vi "NetworkTest.vi"() -> ()   [LabVIEW 2014]
uses:
  <vilib>/Platform/TimedLoop/XDataNode/timing_clust.ctl
  <vilib>/Platform/TimedLoop/XDataNode/nitl_modes.ctl
  <vilib>/Platform/TimedLoop/XDataNode/wakeup.ctl
  <vilib>/Utility/tcp.llb/UDP Multicast Read-Write Open.vi
  <vilib>/platform/TimedLoop/XDataNode/XDataNode.xnode
  <vilib>/Platform/TimedLoop/XDataNode/XDNodeRunTimeDep.lvlib
  <vilib>/Utility/tcp.llb/UDP Multicast Read-Only Open.vi
panel:
  out "address":u32
  out "port":u16
  out "error out":errorcluster
  out "data out 2":string
  out "data out":string
  out "UDP_Out_Error Out 7":errorcluster
  out "UDP_Pack_num 7":u32
  out "UDP_Out Status 7":bool
  in  "Flight Number 5":string
  out "UDP_Out_Error Out 6":errorcluster
  out "UDP_Pack_num 6":u32
  out "UDP_Out Status 6":bool
  in  "Flight Number 4":string
  out "UDP_Out_Error Out 4":errorcluster
  out "UDP_Pack_num 4":u32
  out "UDP_Out Status 4":bool
  in  "Flight Number 3":string
  out "UDP_Out_Error Out 5":errorcluster
  out "UDP_Pack_num 5":u32
  out "UDP_Out Status 5":bool
  in  "Flight Number 2":string
  out "SEPTIC TCP Error Out 5":errorcluster
  out "TCP packet\nSend To SEPTIC 5":bool
  out "FISH TCP Error Out 5":errorcluster
  out "TCP packet\nSend To FISH 5":bool
  out "SEPTIC TCP Error Out 4":errorcluster
  out "TCP packet\nSend To SEPTIC 4":bool
  out "FISH TCP Error Out 4":errorcluster
  out "TCP packet\nSend To FISH 4":bool
  out "SEPTIC TCP Error Out 3":errorcluster
  out "TCP packet\nSend To SEPTIC 3":bool
  out "FISH TCP Error Out 3":errorcluster
  out "TCP packet\nSend To FISH 3":bool
  out "SEPTIC TCP Error Out 2":errorcluster
  out "TCP packet\nSend To SEPTIC 2":bool
  out "FISH TCP Error Out 2":errorcluster
  out "TCP packet\nSend To FISH 2":bool
  out "FISH TCP Error Out":errorcluster
  out "TCP packet\nSend To FISH":bool
  out "SEPTIC TCP Error Out":errorcluster
  out "TCP packet\nSend To SEPTIC":bool
  out "UDP_Pack_num 3":u32
  out "UDP_Out Status 3":bool
  out "UDP_Out_Error Out 3":errorcluster
  out "UDP_In":string
  out "UDP_In_Error":errorcluster
  in  "Flight Number":string
  in  "stop":bool
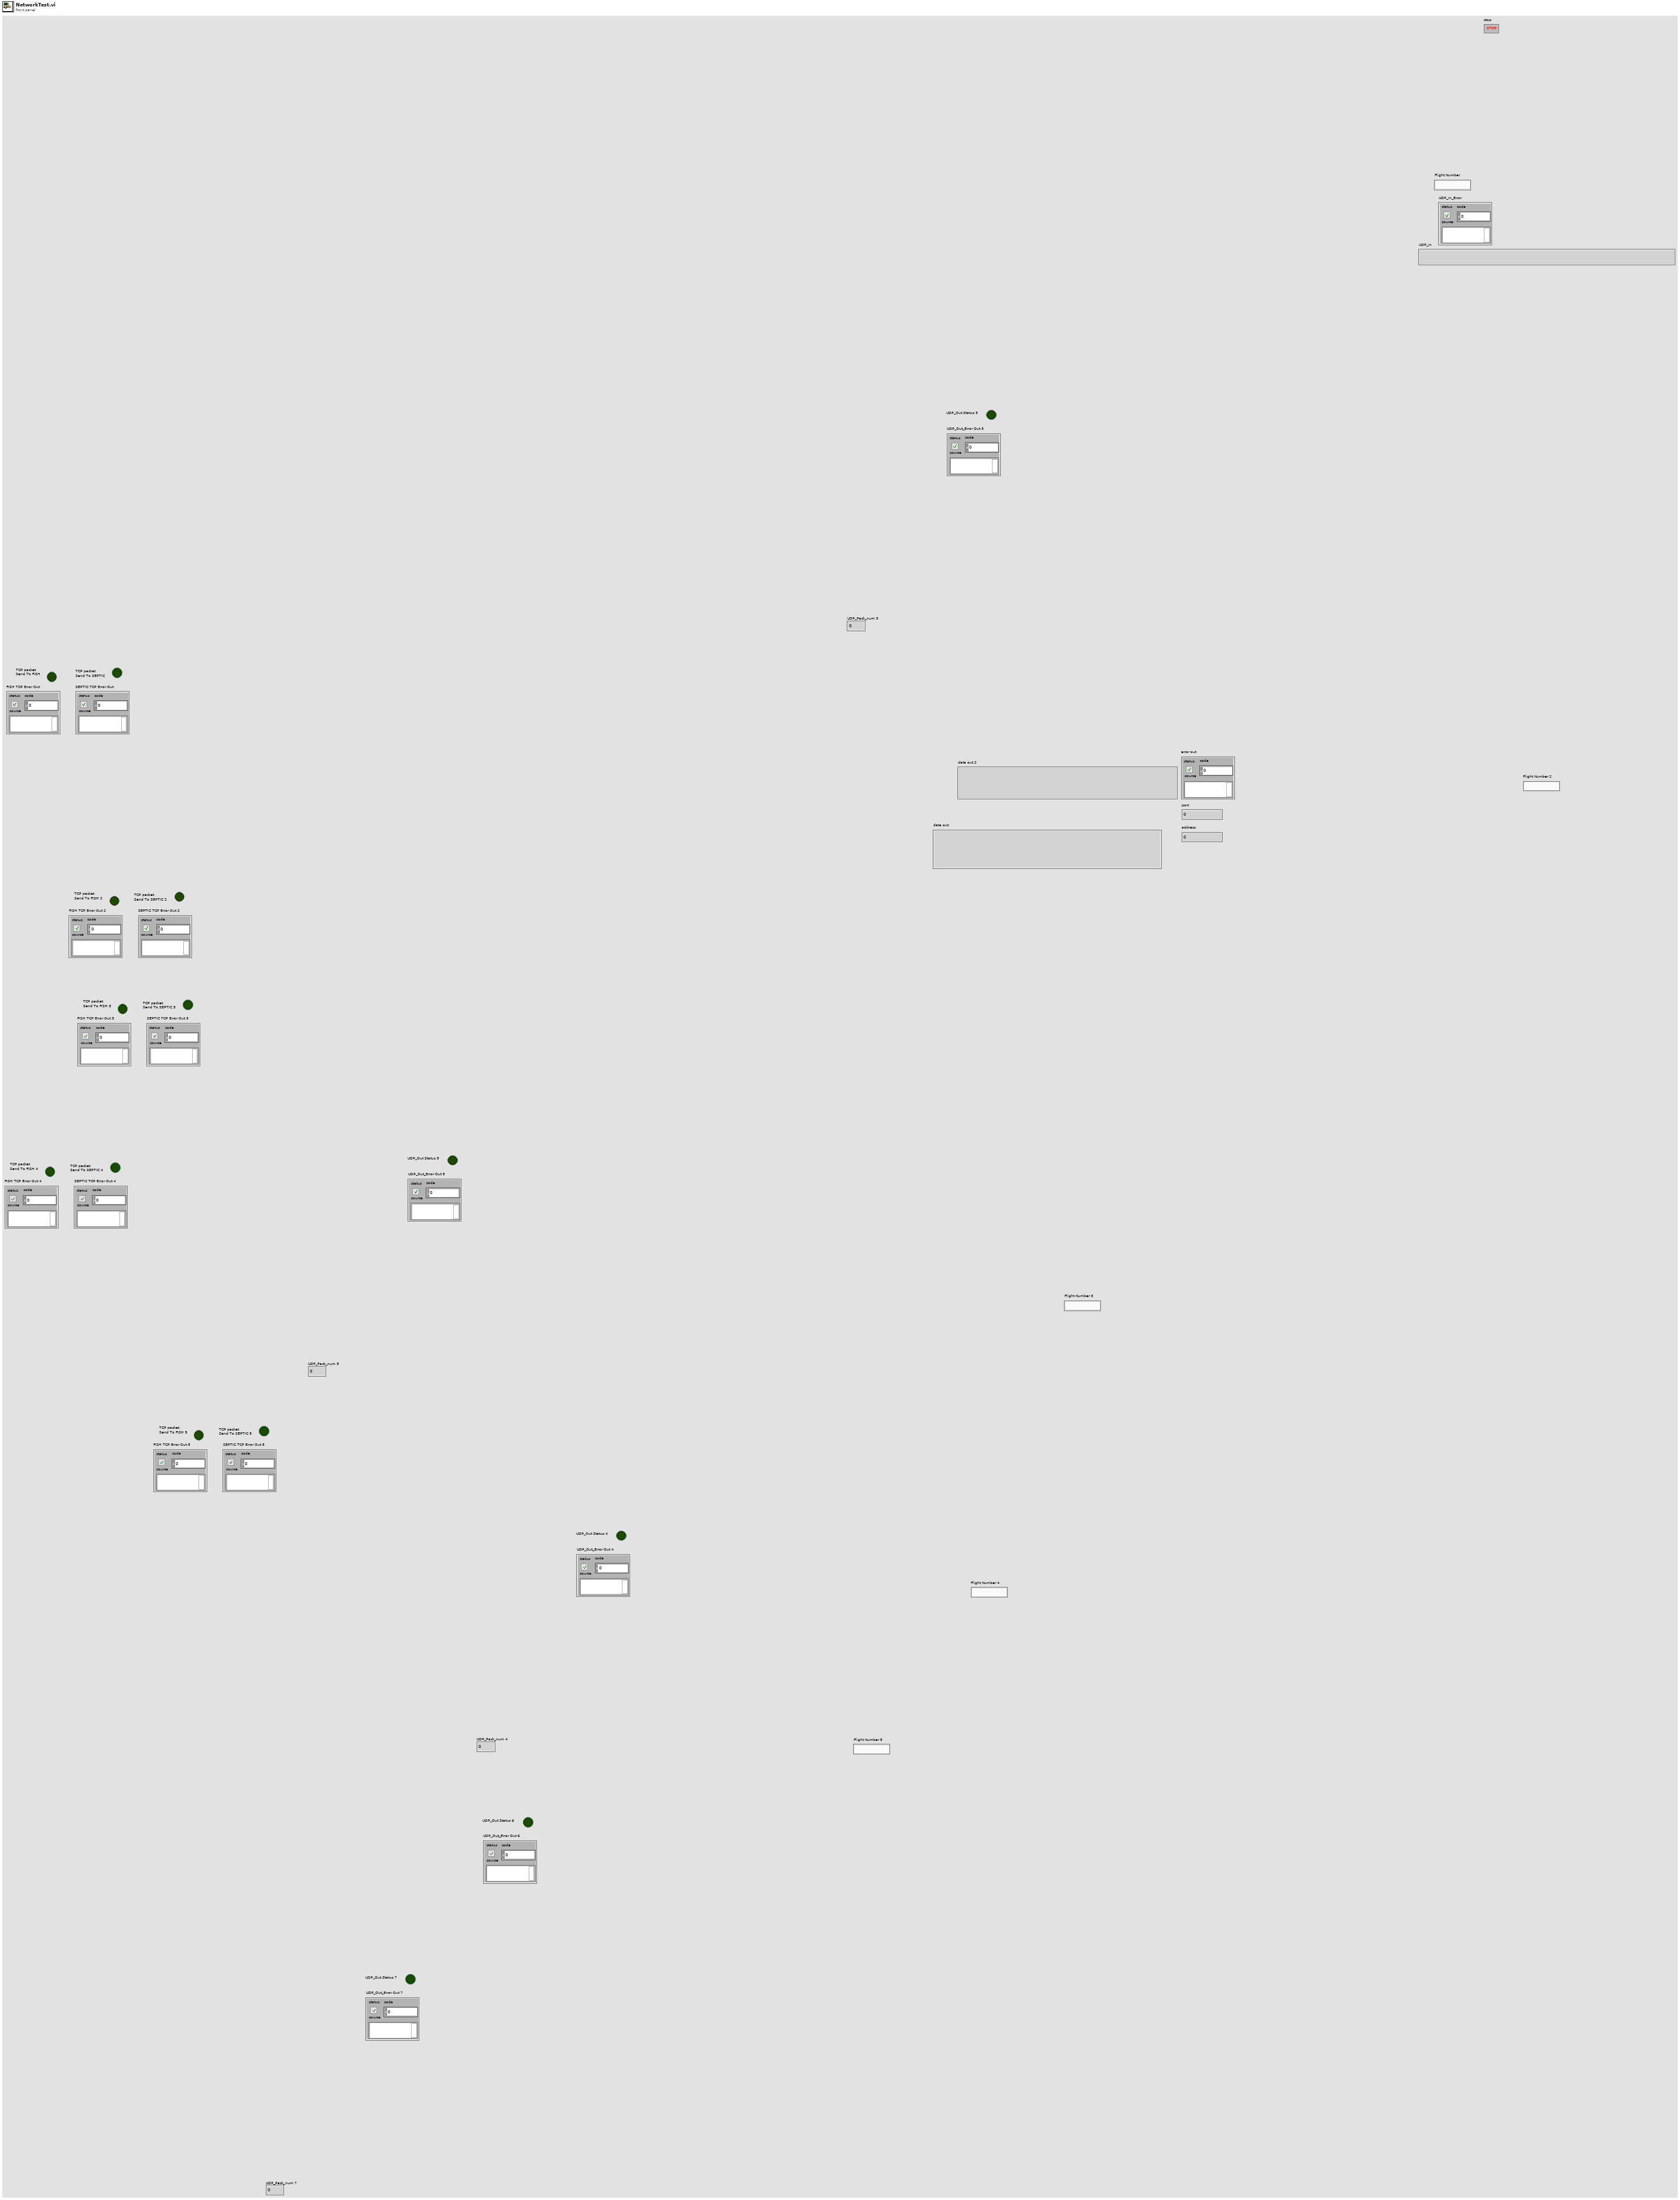
[diagram p1: front panel]
types:
  T1 = typedef "XDNodeRunTimeDep.lvlib/timing_clust.ctl" = cluster{"Expected End [f-1]":u64, "Actual End [f-1]":u64, "Finished Late? [f-1]":bool, "Expected End [i-1]":u64, "Actual End [i-1]":u64, "Finished Late? [i-1]":bool, "Expected Start [i]":u64, "Actual Start [i]":u64, "Expected Start [f]":u64, "Actual Start [f]":u64, "Source Name":string, "Structure Name":string, "Period":i64, "Deadline":i64, "Offset":i64, "Start":i64, "Priority":i32, "Timeout":i32, "Mode":T2, "Wakeup Reason":T3, "Error":errorcluster, "Source Type":string, "Secondary Source Type":string, "Global End Time":u64, "Global Start Time":u64, "Frame Duration":u64, "Iteration Duration":u64, "Assigned CPU":i32, "I/O Scan Engine Mode":u32}
  T2 = typedef "XDNodeRunTimeDep.lvlib/nitl_modes.ctl" = enum32{"No Change", "Process missed periods, maintain original phase", "Discard missed periods, maintain original phase", "Process missed periods, ignore original phase", "Discard missed periods, ignore original phase"}
  T3 = typedef "XDNodeRunTimeDep.lvlib/wakeup.ctl" = enum32{"Normal", "Aborted", "Asynchronous wakeup", "Timing source error", "Timed loop error", "Timeout"}
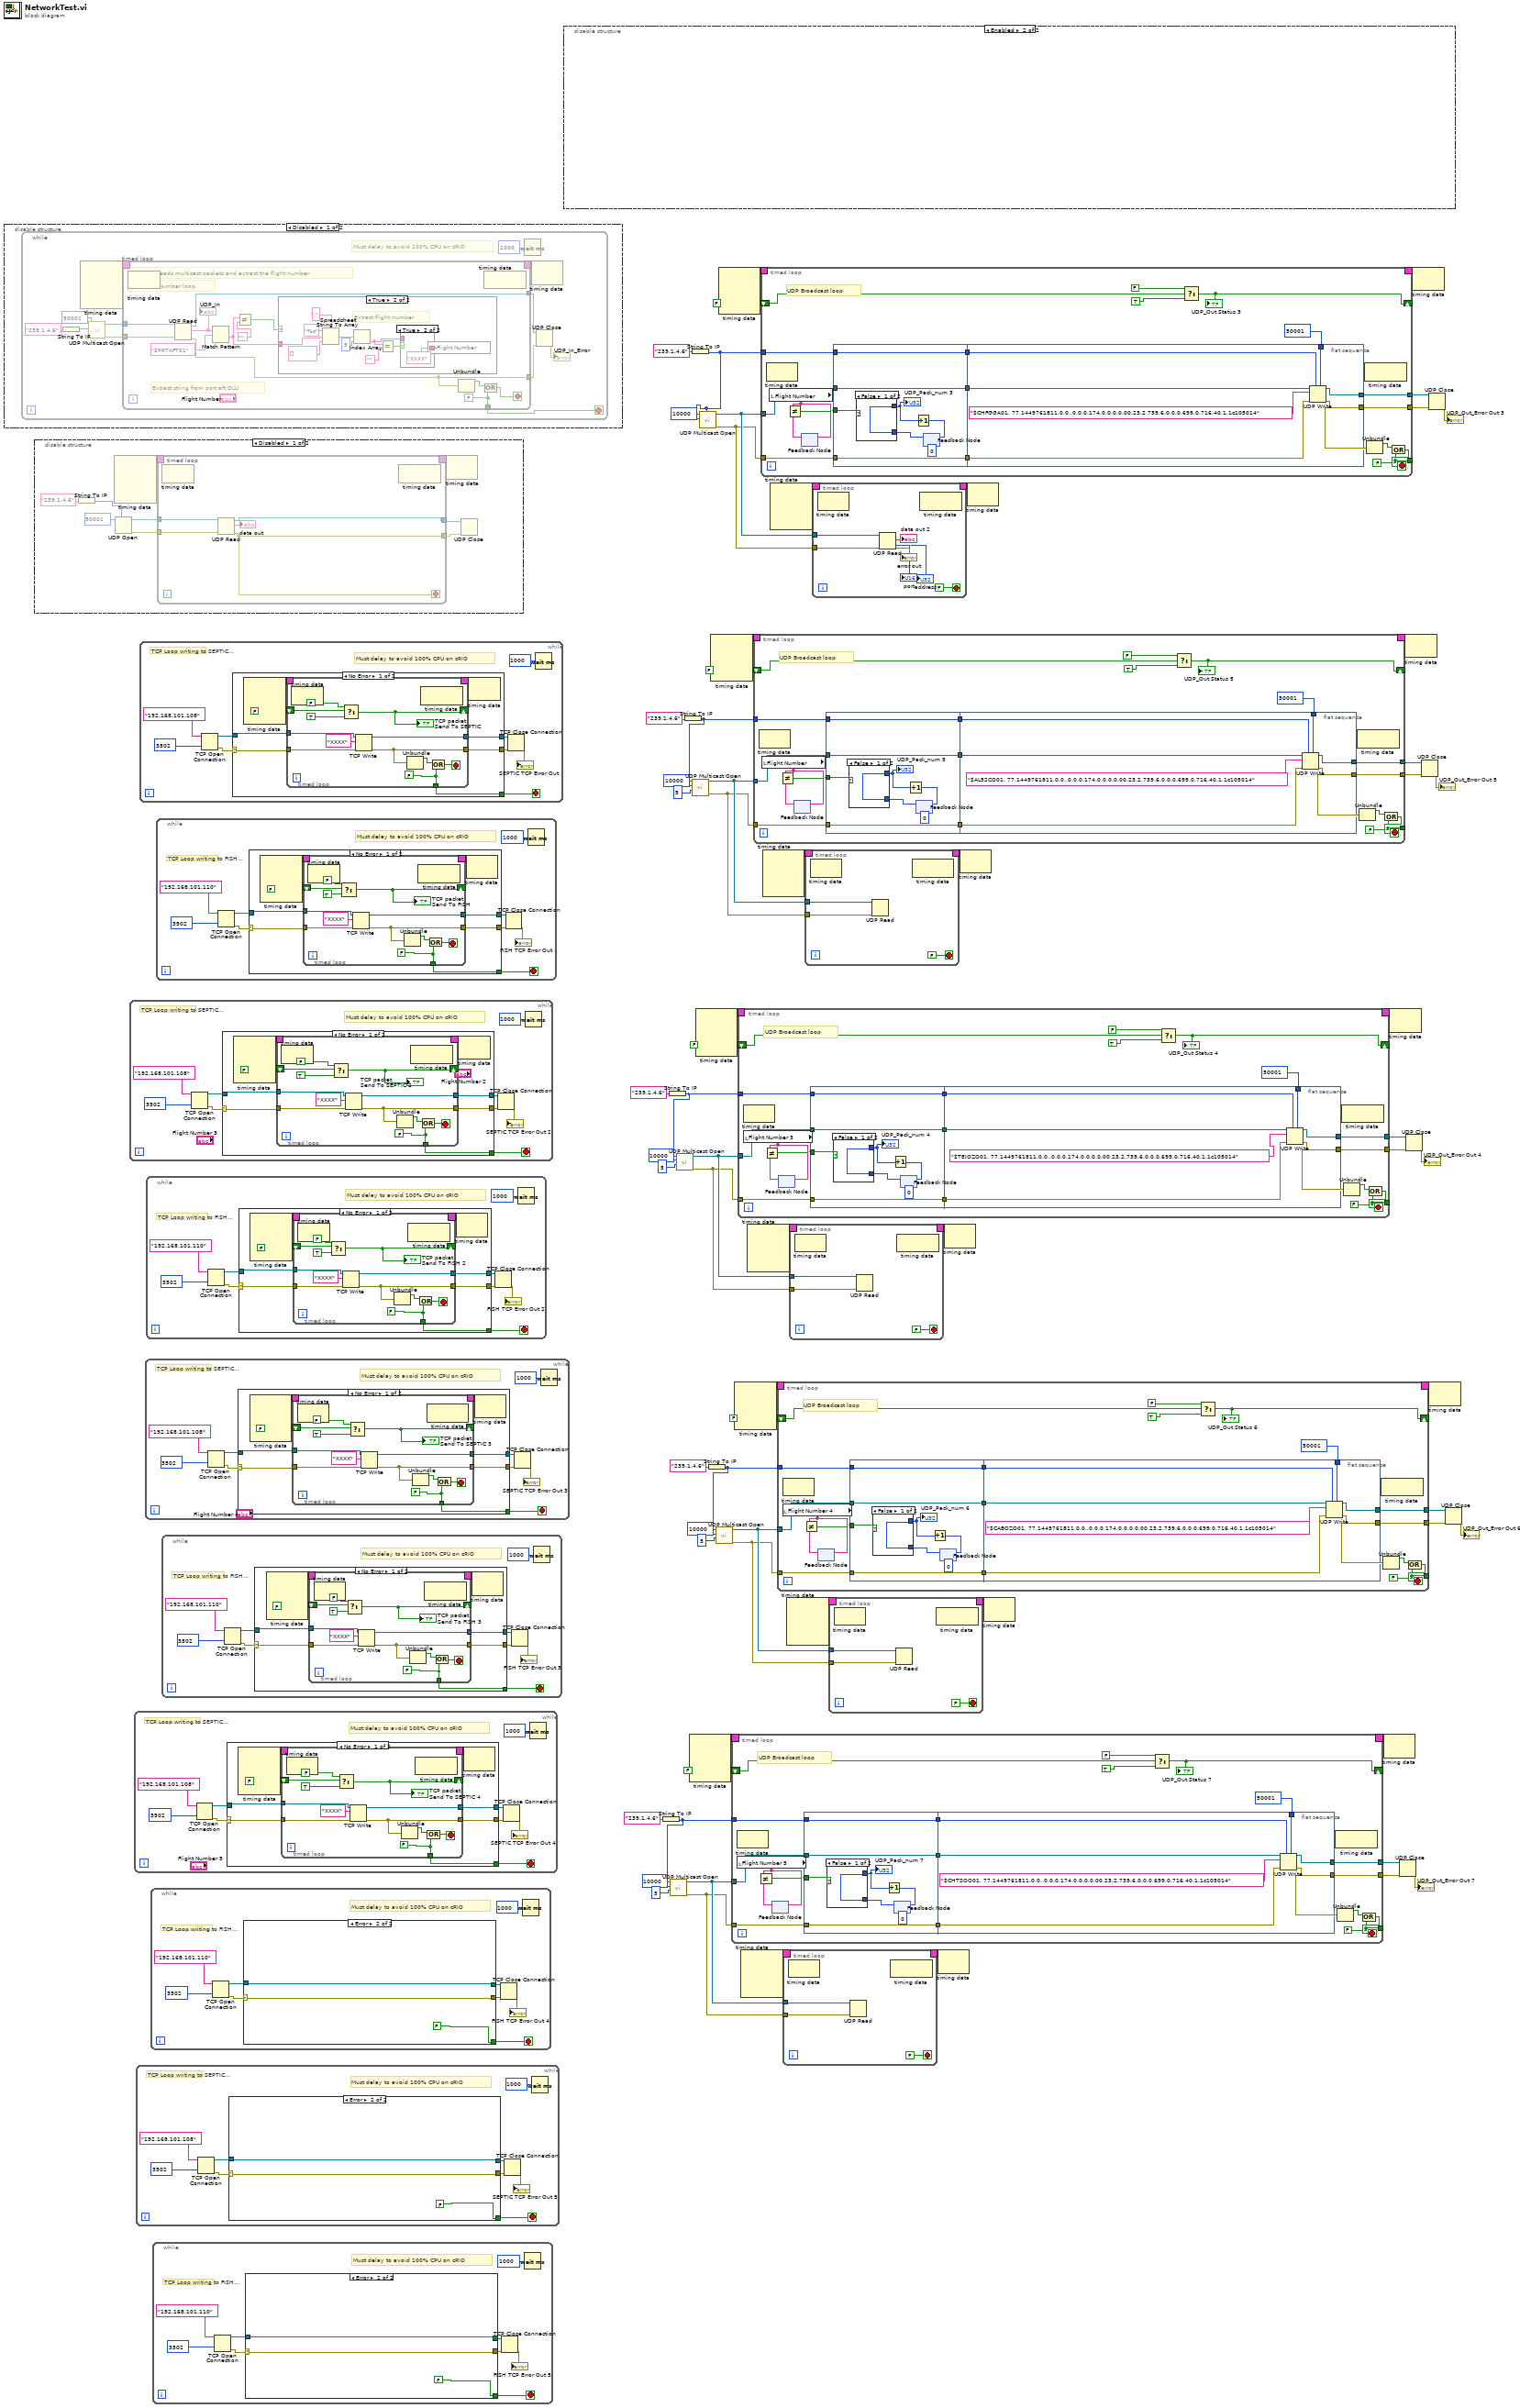
[diagram p0: block diagram]
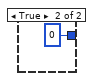
[diagram p6: hidden frame]
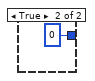
[diagram p7: hidden frame]
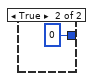
[diagram p8: hidden frame]
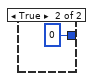
[diagram p9: hidden frame]
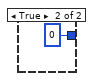
[diagram p10: hidden frame]
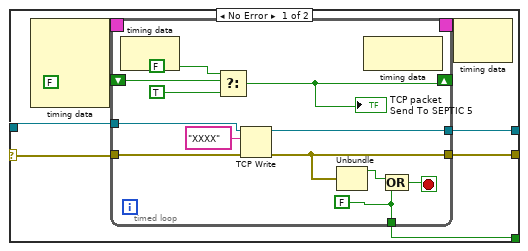
[diagram p11: hidden frame]
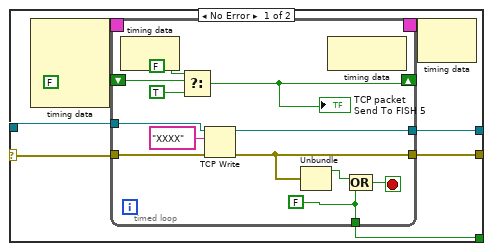
[diagram p12: hidden frame]
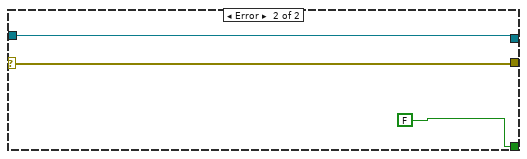
[diagram p13: hidden frame]
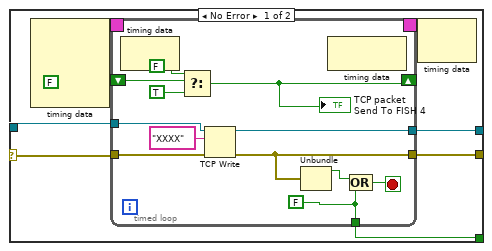
[diagram p14: hidden frame]
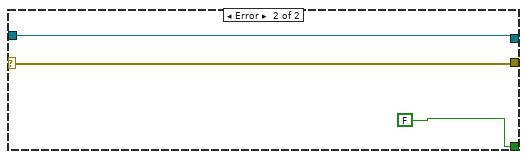
[diagram p15: hidden frame]
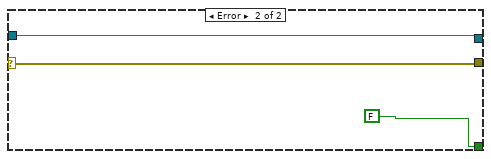
[diagram p16: hidden frame]
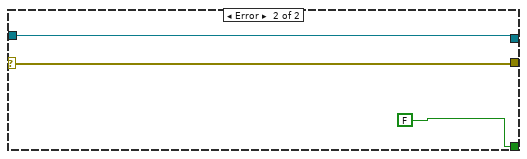
[diagram p17: hidden frame]
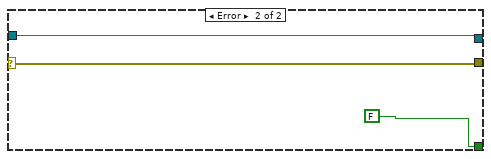
[diagram p18: hidden frame]
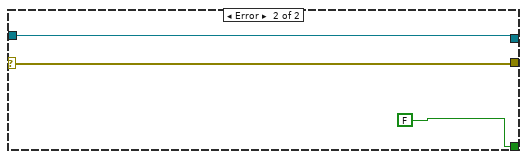
[diagram p19: hidden frame]
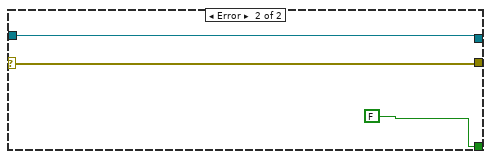
[diagram p20: hidden frame]
diagram:
  n1 = disable-structure shown="Disabled" {
    frame Disabled {
      n2 = while {
        stop <- w71 stop-if-true
        # "Must delay to avoid 100% CPU on cRIO"
        n3 = String To IP(1:"239.1.4.6" ("name")) -> (0:w79:u32)
        n4 = node-c288() -> (w81:T1)  [unwired: 4 in]
        n5 = call-poly <vilib>:"UDP Multicast Open.vi"("multicast addr"=w79, "port"=u16 50001) -> ("error out"=w75:errorcluster, "connection ID"=w76:refnum<k16>)  [unwired: 7 in, 1 out]
        n6 = timed-loop {
          tunnel: w76 -> [w93]
          tunnel: w75 -> [w92]
          timing: w81 -> [_]
          timing-out: [_] -> w80
          tunnel: [w86] -> w73
          tunnel: [w84] -> w72
          tunnel: [w82] -> w71
          stop <- w83 stop-if-true
          w82 = FALSE
          # "Extract string from port aft DLU"
          # "Get Flight Number loop"
          # "This loop reads multicast packets and extract the flight number"
          n7 = node-c288() -> ()  [unwired: 1 in, 1 out]
          n8 = UDP Read(connection ID=w93, 8:w92) -> (data out=w91:string, error out=w84:errorcluster, 3:w86:refnum<k16>)  [unwired: 2 in, 2 out]
          "UDP_In" <- w91
          n9 = Match Pattern(string=w91, regular expression="$PRTAFT01") -> (after substring=w87:string)  [unwired: 1 in, 3 out]
          n10 = Not Equal?(x=w87, y="") -> (x != y?=w88:bool)
          n11 = case shown="True" w88 {
            tunnel: w87 -> [_ w100]
            frame False {
            }
            frame True {
              # "Extract flight number"
              n12 = Spreadsheet String To Array(delimiter (Tab)=",", format string="%s", spreadsheet string=w100, array type (2D Dbl)=string[] []) -> (array=w102:string[])
              n13 = Index Array(array=w102, index=5) -> (element=w96:string)
              n14 = Equal?(x=w96, y="") -> (x = y?=w99:bool)
              n15 = case shown="True" w99 {
                tunnel: [w106 "XXXX"] -> w97
                tunnel: w96 -> [w106 _]
                frame False {
                }
                frame True {
                }
              }
              n16 = local write "Flight Number"(w97) -> ()
            }
          }
          n17 = Unbundle(w84) -> ("status"=w85:bool)  [unwired: 2 out]
          n18 = node-c288() -> ()  [unwired: 1 in, 1 out]
          n19 = Compound Arithmetic op=OR(w85, w82) -> (w83:bool)
        }
        n20 = Wait (ms)(milliseconds to wait=u32 1000) -> ()  [unwired: 1 out]
        n21 = node-c288(w80) -> ()  [unwired: 1 out]
        n22 = UDP Close(connection ID=w73, 8:w72) -> (error out=→"UDP_In_Error":errorcluster)  [unwired: 1 out]
      }
    }
    frame Enabled {
    }
  }
  n23 = disable-structure shown="Disabled" {
    frame Disabled {
      n24 = String To IP(1:"239.1.4.6" ("name")) -> (0:w110:u32)
      n25 = node-c288() -> (w118:T1)  [unwired: 4 in]
      n26 = UDP Open(7:w110, 11:u16 50001 ("port")) -> (port=w115:refnum<k16>, 0:w114:errorcluster)  [unwired: 3 in, 1 out]
      n27 = timed-loop {
        timing: w118 -> [_]
        timing-out: [_] -> w117
        tunnel: w115 -> [w123]
        tunnel: w114 -> [w122]
        tunnel: [w120] -> w112
        tunnel: [w119] -> w113
        stop <- w120 stop-if-true
        n28 = node-c288() -> ()  [unwired: 1 in, 1 out]
        n29 = UDP Read(connection ID=w123, 8:w122) -> (data out=→"data out":string, error out=w120:errorcluster, 3:w119:refnum<k16>)  [unwired: 2 in, 2 out]
        n30 = node-c288() -> ()  [unwired: 1 in, 1 out]
      }
      n31 = node-c288(w117) -> ()  [unwired: 1 out]
      n32 = UDP Close(connection ID=w113, 8:w112) -> ()  [unwired: 2 out]
    }
    frame Enabled {
    }
  }
  n33 = while {
    stop <- w131 stop-if-true
    # "Must delay to avoid 100% CPU on cRIO"
    # "TCP Loop writing to SEPTIC Tank"
    n34 = TCP Open Connection(address="192.168.101.108", remote port or service name=u16 3502) -> (connection ID=w134:refnum<k5>, error out=w129:errorcluster)  [unwired: 3 in]
    n35 = case shown="No Error" w129 {
      selector: w129 -> [w137 w162]
      tunnel: w134 -> [w142 w163]
      tunnel: [w141 w163] -> w133
      tunnel: [w140 w162] -> w132
      tunnel: [w139 FALSE] -> w131
      frame No Error {
        n36 = node-c288() -> (w144:T1)  [unwired: 4 in]
        n37 = timed-loop {
          tunnel: w142 -> [w156]
          tunnel: w137 -> [w155]
          tunnel: [w154] -> w141
          tunnel: [w153] -> w140
          tunnel: [w146] -> w139
          shift-right: [w147] -> _
          shift-left: FALSE -> [w150]
          timing: w144 -> [_]
          timing-out: [_] -> w143
          stop <- w151 stop-if-true
          w146 = FALSE
          n38 = node-c288() -> ()  [unwired: 1 in, 1 out]
          n39 = Select(t=FALSE, s=w150, f=TRUE) -> (s? t:f=w147:bool)
          "TCP packet\nSend To SEPTIC 2" <- w147
          n40 = TCP Write(connection ID=w156, data in="XXXX", error in (no error)=w155) -> (connection ID out=w154:refnum<k5>, error out=w153:errorcluster)  [unwired: 1 in, 1 out]
          n41 = Unbundle(w153) -> ("status"=w152:bool)  [unwired: 2 out]
          n42 = node-c288() -> ()  [unwired: 1 in, 1 out]
          n43 = Compound Arithmetic op=OR(w152, w146) -> (w151:bool)
        }
        n44 = node-c288(w143) -> ()  [unwired: 1 out]
      }
      frame Error {
      }
    }
    n45 = TCP Close Connection(connection ID=w133, error in (no error)=w132) -> (error out=→"SEPTIC TCP Error Out 2":errorcluster)  [unwired: 1 in, 1 out]
    n46 = Wait (ms)(milliseconds to wait=u32 1000) -> ()  [unwired: 1 out]
  }
  n47 = while {
    stop <- w167 stop-if-true
    # "Must delay to avoid 100% CPU on cRIO"
    # "TCP Loop writing to SEPTIC Tank"
    n48 = TCP Open Connection(address="192.168.101.108", remote port or service name=u16 3502) -> (connection ID=w170:refnum<k5>, error out=w165:errorcluster)  [unwired: 3 in]
    n49 = case shown="No Error" w165 {
      selector: w165 -> [w173 w198]
      tunnel: w170 -> [w178 w199]
      tunnel: [w177 w199] -> w169
      tunnel: [w176 w198] -> w168
      tunnel: [w175 FALSE] -> w167
      frame No Error {
        n50 = node-c288() -> (w180:T1)  [unwired: 4 in]
        n51 = timed-loop {
          tunnel: w178 -> [w192]
          tunnel: w173 -> [w191]
          tunnel: [w190] -> w177
          tunnel: [w189] -> w176
          tunnel: [w182] -> w175
          shift-right: [w183] -> _
          shift-left: FALSE -> [w186]
          timing: w180 -> [_]
          timing-out: [_] -> w179
          stop <- w187 stop-if-true
          w182 = FALSE
          n52 = node-c288() -> ()  [unwired: 1 in, 1 out]
          n53 = Select(t=FALSE, s=w186, f=TRUE) -> (s? t:f=w183:bool)
          "TCP packet\nSend To SEPTIC 4" <- w183
          n54 = TCP Write(connection ID=w192, data in="XXXX", error in (no error)=w191) -> (connection ID out=w190:refnum<k5>, error out=w189:errorcluster)  [unwired: 1 in, 1 out]
          n55 = Unbundle(w189) -> ("status"=w188:bool)  [unwired: 2 out]
          n56 = node-c288() -> ()  [unwired: 1 in, 1 out]
          n57 = Compound Arithmetic op=OR(w188, w182) -> (w187:bool)
        }
        n58 = node-c288(w179) -> ()  [unwired: 1 out]
      }
      frame Error {
      }
    }
    n59 = TCP Close Connection(connection ID=w169, error in (no error)=w168) -> (error out=→"SEPTIC TCP Error Out 4":errorcluster)  [unwired: 1 in, 1 out]
    n60 = Wait (ms)(milliseconds to wait=u32 1000) -> ()  [unwired: 1 out]
  }
  n61 = while {
    stop <- w203 stop-if-true
    # "Must delay to avoid 100% CPU on cRIO"
    # "TCP Loop writing to SEPTIC Tank"
    n62 = TCP Open Connection(address="192.168.101.108", remote port or service name=u16 3502) -> (connection ID=w206:refnum<k5>, error out=w201:errorcluster)  [unwired: 3 in]
    n63 = case shown="Error" w201 {
      selector: w201 -> [w209 w234]
      tunnel: w206 -> [w214 w235]
      tunnel: [w213 w235] -> w205
      tunnel: [w212 w234] -> w204
      tunnel: [w211 FALSE] -> w203
      frame No Error {
        n64 = node-c288() -> (w216:T1)  [unwired: 4 in]
        n65 = timed-loop {
          tunnel: w214 -> [w228]
          tunnel: w209 -> [w227]
          tunnel: [w226] -> w213
          tunnel: [w225] -> w212
          tunnel: [w218] -> w211
          shift-right: [w219] -> _
          shift-left: FALSE -> [w222]
          timing: w216 -> [_]
          timing-out: [_] -> w215
          stop <- w223 stop-if-true
          w218 = FALSE
          n66 = node-c288() -> ()  [unwired: 1 in, 1 out]
          n67 = Select(t=FALSE, s=w222, f=TRUE) -> (s? t:f=w219:bool)
          "TCP packet\nSend To SEPTIC 5" <- w219
          n68 = TCP Write(connection ID=w228, data in="XXXX", error in (no error)=w227) -> (connection ID out=w226:refnum<k5>, error out=w225:errorcluster)  [unwired: 1 in, 1 out]
          n69 = Unbundle(w225) -> ("status"=w224:bool)  [unwired: 2 out]
          n70 = node-c288() -> ()  [unwired: 1 in, 1 out]
          n71 = Compound Arithmetic op=OR(w224, w218) -> (w223:bool)
        }
        n72 = node-c288(w215) -> ()  [unwired: 1 out]
      }
      frame Error {
      }
    }
    n73 = TCP Close Connection(connection ID=w205, error in (no error)=w204) -> (error out=→"SEPTIC TCP Error Out 5":errorcluster)  [unwired: 1 in, 1 out]
    n74 = Wait (ms)(milliseconds to wait=u32 1000) -> ()  [unwired: 1 out]
  }
  n75 = while {
    stop <- w239 stop-if-true
    # "Must delay to avoid 100% CPU on cRIO"
    # "TCP Loop writing to SEPTIC Tank"
    n76 = TCP Open Connection(address="192.168.101.108", remote port or service name=u16 3502) -> (connection ID=w242:refnum<k5>, error out=w237:errorcluster)  [unwired: 3 in]
    n77 = case shown="No Error" w237 {
      selector: w237 -> [w245 w270]
      tunnel: w242 -> [w250 w271]
      tunnel: [w249 w271] -> w241
      tunnel: [w248 w270] -> w240
      tunnel: [w247 FALSE] -> w239
      frame No Error {
        n78 = node-c288() -> (w252:T1)  [unwired: 4 in]
        n79 = timed-loop {
          tunnel: w250 -> [w264]
          tunnel: w245 -> [w263]
          tunnel: [w262] -> w249
          tunnel: [w261] -> w248
          tunnel: [w254] -> w247
          shift-right: [w255] -> _
          shift-left: FALSE -> [w258]
          timing: w252 -> [_]
          timing-out: [_] -> w251
          stop <- w259 stop-if-true
          w254 = FALSE
          n80 = node-c288() -> ()  [unwired: 1 in, 1 out]
          n81 = Select(t=FALSE, s=w258, f=TRUE) -> (s? t:f=w255:bool)
          "TCP packet\nSend To SEPTIC" <- w255
          n82 = TCP Write(connection ID=w264, data in="XXXX", error in (no error)=w263) -> (connection ID out=w262:refnum<k5>, error out=w261:errorcluster)  [unwired: 1 in, 1 out]
          n83 = Unbundle(w261) -> ("status"=w260:bool)  [unwired: 2 out]
          n84 = node-c288() -> ()  [unwired: 1 in, 1 out]
          n85 = Compound Arithmetic op=OR(w260, w254) -> (w259:bool)
        }
        n86 = node-c288(w251) -> ()  [unwired: 1 out]
      }
      frame Error {
      }
    }
    n87 = TCP Close Connection(connection ID=w241, error in (no error)=w240) -> (error out=→"SEPTIC TCP Error Out":errorcluster)  [unwired: 1 in, 1 out]
    n88 = Wait (ms)(milliseconds to wait=u32 1000) -> ()  [unwired: 1 out]
  }
  n89 = while {
    stop <- w275 stop-if-true
    # "Must delay to avoid 100% CPU on cRIO"
    # "TCP Loop writing to SEPTIC Tank"
    n90 = TCP Open Connection(address="192.168.101.108", remote port or service name=u16 3502) -> (connection ID=w278:refnum<k5>, error out=w273:errorcluster)  [unwired: 3 in]
    n91 = case shown="No Error" w273 {
      selector: w273 -> [w281 w306]
      tunnel: w278 -> [w286 w307]
      tunnel: [w285 w307] -> w277
      tunnel: [w284 w306] -> w276
      tunnel: [w283 FALSE] -> w275
      frame No Error {
        n92 = node-c288() -> (w288:T1)  [unwired: 4 in]
        n93 = timed-loop {
          tunnel: w286 -> [w300]
          tunnel: w281 -> [w299]
          tunnel: [w298] -> w285
          tunnel: [w297] -> w284
          tunnel: [w290] -> w283
          shift-right: [w291] -> _
          shift-left: FALSE -> [w294]
          timing: w288 -> [_]
          timing-out: [_] -> w287
          stop <- w295 stop-if-true
          w290 = FALSE
          n94 = node-c288() -> ()  [unwired: 1 in, 1 out]
          n95 = Select(t=FALSE, s=w294, f=TRUE) -> (s? t:f=w291:bool)
          "TCP packet\nSend To SEPTIC 3" <- w291
          n96 = TCP Write(connection ID=w300, data in="XXXX", error in (no error)=w299) -> (connection ID out=w298:refnum<k5>, error out=w297:errorcluster)  [unwired: 1 in, 1 out]
          n97 = Unbundle(w297) -> ("status"=w296:bool)  [unwired: 2 out]
          n98 = node-c288() -> ()  [unwired: 1 in, 1 out]
          n99 = Compound Arithmetic op=OR(w296, w290) -> (w295:bool)
        }
        n100 = node-c288(w287) -> ()  [unwired: 1 out]
      }
      frame Error {
      }
    }
    n101 = TCP Close Connection(connection ID=w277, error in (no error)=w276) -> (error out=→"SEPTIC TCP Error Out 3":errorcluster)  [unwired: 1 in, 1 out]
    n102 = Wait (ms)(milliseconds to wait=u32 1000) -> ()  [unwired: 1 out]
  }
  n103 = while {
    stop <- w311 stop-if-true
    # "Must delay to avoid 100% CPU on cRIO"
    # "TCP Loop writing to FISH Tank"
    n104 = TCP Open Connection(address="192.168.101.110", remote port or service name=u16 3502) -> (connection ID=w314:refnum<k5>, error out=w309:errorcluster)  [unwired: 3 in]
    n105 = case shown="No Error" w309 {
      selector: w309 -> [w317 w342]
      tunnel: w314 -> [w322 w343]
      tunnel: [w321 w343] -> w313
      tunnel: [w320 w342] -> w312
      tunnel: [w319 FALSE] -> w311
      frame No Error {
        n106 = node-c288() -> (w324:T1)  [unwired: 4 in]
        n107 = timed-loop {
          tunnel: w322 -> [w336]
          tunnel: w317 -> [w335]
          tunnel: [w334] -> w321
          tunnel: [w333] -> w320
          tunnel: [w326] -> w319
          shift-right: [w327] -> _
          shift-left: FALSE -> [w330]
          timing: w324 -> [_]
          timing-out: [_] -> w323
          stop <- w331 stop-if-true
          w326 = FALSE
          n108 = node-c288() -> ()  [unwired: 1 in, 1 out]
          n109 = Select(t=FALSE, s=w330, f=TRUE) -> (s? t:f=w327:bool)
          "TCP packet\nSend To FISH 2" <- w327
          n110 = TCP Write(connection ID=w336, data in="XXXX", error in (no error)=w335) -> (connection ID out=w334:refnum<k5>, error out=w333:errorcluster)  [unwired: 1 in, 1 out]
          n111 = Unbundle(w333) -> ("status"=w332:bool)  [unwired: 2 out]
          n112 = node-c288() -> ()  [unwired: 1 in, 1 out]
          n113 = Compound Arithmetic op=OR(w332, w326) -> (w331:bool)
        }
        n114 = node-c288(w323) -> ()  [unwired: 1 out]
      }
      frame Error {
      }
    }
    n115 = TCP Close Connection(connection ID=w313, error in (no error)=w312) -> (error out=→"FISH TCP Error Out 2":errorcluster)  [unwired: 1 in, 1 out]
    n116 = Wait (ms)(milliseconds to wait=u32 1000) -> ()  [unwired: 1 out]
  }
  n117 = while {
    stop <- w347 stop-if-true
    # "Must delay to avoid 100% CPU on cRIO"
    # "TCP Loop writing to FISH Tank"
    n118 = TCP Open Connection(address="192.168.101.110", remote port or service name=u16 3502) -> (connection ID=w350:refnum<k5>, error out=w345:errorcluster)  [unwired: 3 in]
    n119 = case shown="Error" w345 {
      selector: w345 -> [w353 w378]
      tunnel: w350 -> [w358 w379]
      tunnel: [w357 w379] -> w349
      tunnel: [w356 w378] -> w348
      tunnel: [w355 FALSE] -> w347
      frame No Error {
        n120 = node-c288() -> (w360:T1)  [unwired: 4 in]
        n121 = timed-loop {
          tunnel: w358 -> [w372]
          tunnel: w353 -> [w371]
          tunnel: [w370] -> w357
          tunnel: [w369] -> w356
          tunnel: [w362] -> w355
          shift-right: [w363] -> _
          shift-left: FALSE -> [w366]
          timing: w360 -> [_]
          timing-out: [_] -> w359
          stop <- w367 stop-if-true
          w362 = FALSE
          n122 = node-c288() -> ()  [unwired: 1 in, 1 out]
          n123 = Select(t=FALSE, s=w366, f=TRUE) -> (s? t:f=w363:bool)
          "TCP packet\nSend To FISH 4" <- w363
          n124 = TCP Write(connection ID=w372, data in="XXXX", error in (no error)=w371) -> (connection ID out=w370:refnum<k5>, error out=w369:errorcluster)  [unwired: 1 in, 1 out]
          n125 = Unbundle(w369) -> ("status"=w368:bool)  [unwired: 2 out]
          n126 = node-c288() -> ()  [unwired: 1 in, 1 out]
          n127 = Compound Arithmetic op=OR(w368, w362) -> (w367:bool)
        }
        n128 = node-c288(w359) -> ()  [unwired: 1 out]
      }
      frame Error {
      }
    }
    n129 = TCP Close Connection(connection ID=w349, error in (no error)=w348) -> (error out=→"FISH TCP Error Out 4":errorcluster)  [unwired: 1 in, 1 out]
    n130 = Wait (ms)(milliseconds to wait=u32 1000) -> ()  [unwired: 1 out]
  }
  n131 = while {
    stop <- w383 stop-if-true
    # "Must delay to avoid 100% CPU on cRIO"
    # "TCP Loop writing to FISH Tank"
    n132 = TCP Open Connection(address="192.168.101.110", remote port or service name=u16 3502) -> (connection ID=w386:refnum<k5>, error out=w381:errorcluster)  [unwired: 3 in]
    n133 = case shown="Error" w381 {
      selector: w381 -> [w389 w414]
      tunnel: w386 -> [w394 w415]
      tunnel: [w393 w415] -> w385
      tunnel: [w392 w414] -> w384
      tunnel: [w391 FALSE] -> w383
      frame No Error {
        n134 = node-c288() -> (w396:T1)  [unwired: 4 in]
        n135 = timed-loop {
          tunnel: w394 -> [w408]
          tunnel: w389 -> [w407]
          tunnel: [w406] -> w393
          tunnel: [w405] -> w392
          tunnel: [w398] -> w391
          shift-right: [w399] -> _
          shift-left: FALSE -> [w402]
          timing: w396 -> [_]
          timing-out: [_] -> w395
          stop <- w403 stop-if-true
          w398 = FALSE
          n136 = node-c288() -> ()  [unwired: 1 in, 1 out]
          n137 = Select(t=FALSE, s=w402, f=TRUE) -> (s? t:f=w399:bool)
          "TCP packet\nSend To FISH 5" <- w399
          n138 = TCP Write(connection ID=w408, data in="XXXX", error in (no error)=w407) -> (connection ID out=w406:refnum<k5>, error out=w405:errorcluster)  [unwired: 1 in, 1 out]
          n139 = Unbundle(w405) -> ("status"=w404:bool)  [unwired: 2 out]
          n140 = node-c288() -> ()  [unwired: 1 in, 1 out]
          n141 = Compound Arithmetic op=OR(w404, w398) -> (w403:bool)
        }
        n142 = node-c288(w395) -> ()  [unwired: 1 out]
      }
      frame Error {
      }
    }
    n143 = TCP Close Connection(connection ID=w385, error in (no error)=w384) -> (error out=→"FISH TCP Error Out 5":errorcluster)  [unwired: 1 in, 1 out]
    n144 = Wait (ms)(milliseconds to wait=u32 1000) -> ()  [unwired: 1 out]
  }
  n145 = while {
    stop <- w419 stop-if-true
    # "Must delay to avoid 100% CPU on cRIO"
    # "TCP Loop writing to FISH Tank"
    n146 = TCP Open Connection(address="192.168.101.110", remote port or service name=u16 3502) -> (connection ID=w422:refnum<k5>, error out=w417:errorcluster)  [unwired: 3 in]
    n147 = case shown="No Error" w417 {
      selector: w417 -> [w425 w450]
      tunnel: w422 -> [w430 w451]
      tunnel: [w429 w451] -> w421
      tunnel: [w428 w450] -> w420
      tunnel: [w427 FALSE] -> w419
      frame No Error {
        n148 = node-c288() -> (w432:T1)  [unwired: 4 in]
        n149 = timed-loop {
          tunnel: w430 -> [w444]
          tunnel: w425 -> [w443]
          tunnel: [w442] -> w429
          tunnel: [w441] -> w428
          tunnel: [w434] -> w427
          shift-right: [w435] -> _
          shift-left: FALSE -> [w438]
          timing: w432 -> [_]
          timing-out: [_] -> w431
          stop <- w439 stop-if-true
          w434 = FALSE
          n150 = node-c288() -> ()  [unwired: 1 in, 1 out]
          n151 = Select(t=FALSE, s=w438, f=TRUE) -> (s? t:f=w435:bool)
          "TCP packet\nSend To FISH" <- w435
          n152 = TCP Write(connection ID=w444, data in="XXXX", error in (no error)=w443) -> (connection ID out=w442:refnum<k5>, error out=w441:errorcluster)  [unwired: 1 in, 1 out]
          n153 = Unbundle(w441) -> ("status"=w440:bool)  [unwired: 2 out]
          n154 = node-c288() -> ()  [unwired: 1 in, 1 out]
          n155 = Compound Arithmetic op=OR(w440, w434) -> (w439:bool)
        }
        n156 = node-c288(w431) -> ()  [unwired: 1 out]
      }
      frame Error {
      }
    }
    n157 = TCP Close Connection(connection ID=w421, error in (no error)=w420) -> (error out=→"FISH TCP Error Out":errorcluster)  [unwired: 1 in, 1 out]
    n158 = Wait (ms)(milliseconds to wait=u32 1000) -> ()  [unwired: 1 out]
  }
  n159 = while {
    stop <- w455 stop-if-true
    # "Must delay to avoid 100% CPU on cRIO"
    # "TCP Loop writing to FISH Tank"
    n160 = TCP Open Connection(address="192.168.101.110", remote port or service name=u16 3502) -> (connection ID=w458:refnum<k5>, error out=w453:errorcluster)  [unwired: 3 in]
    n161 = case shown="No Error" w453 {
      selector: w453 -> [w461 w486]
      tunnel: w458 -> [w466 w487]
      tunnel: [w465 w487] -> w457
      tunnel: [w464 w486] -> w456
      tunnel: [w463 FALSE] -> w455
      frame No Error {
        n162 = node-c288() -> (w468:T1)  [unwired: 4 in]
        n163 = timed-loop {
          tunnel: w466 -> [w480]
          tunnel: w461 -> [w479]
          tunnel: [w478] -> w465
          tunnel: [w477] -> w464
          tunnel: [w470] -> w463
          shift-right: [w471] -> _
          shift-left: FALSE -> [w474]
          timing: w468 -> [_]
          timing-out: [_] -> w467
          stop <- w475 stop-if-true
          w470 = FALSE
          n164 = node-c288() -> ()  [unwired: 1 in, 1 out]
          n165 = Select(t=FALSE, s=w474, f=TRUE) -> (s? t:f=w471:bool)
          "TCP packet\nSend To FISH 3" <- w471
          n166 = TCP Write(connection ID=w480, data in="XXXX", error in (no error)=w479) -> (connection ID out=w478:refnum<k5>, error out=w477:errorcluster)  [unwired: 1 in, 1 out]
          n167 = Unbundle(w477) -> ("status"=w476:bool)  [unwired: 2 out]
          n168 = node-c288() -> ()  [unwired: 1 in, 1 out]
          n169 = Compound Arithmetic op=OR(w476, w470) -> (w475:bool)
        }
        n170 = node-c288(w467) -> ()  [unwired: 1 out]
      }
      frame Error {
      }
    }
    n171 = TCP Close Connection(connection ID=w457, error in (no error)=w456) -> (error out=→"FISH TCP Error Out 3":errorcluster)  [unwired: 1 in, 1 out]
    n172 = Wait (ms)(milliseconds to wait=u32 1000) -> ()  [unwired: 1 out]
  }
  n173 = disable-structure shown="Enabled" {
    frame Disabled {
      n174 = String To IP(1:"192.168.101.17") -> (0:w488:u32)
      n175 = UDP Open(7:w488) -> (port=w493:refnum<k16>, 0:w492:errorcluster)  [unwired: 4 in, 1 out]
      n176 = while {
        shift-right: [w496] -> w491
        shift-left: w493 -> [w499]
        shift-right: [w495] -> w490
        shift-left: w492 -> [w498]
        stop <- "stop" stop-if-true
        n177 = UDP Write(connection ID=w499, 8:w498) -> (data in=w497:string, error out=w495:errorcluster, 3:w496:refnum<k16>)  [unwired: 3 in]
      }
      n178 = UDP Close(connection ID=w491, 8:w490) -> ()  [unwired: 2 out]
    }
    frame Enabled {
    }
  }
  n179 = String To IP(1:"239.1.4.6" ("name")) -> (0:w2:u32)
  n180 = String To IP(1:"239.1.4.6" ("name")) -> (0:w30:u32)
  n181 = call-poly <vilib>:"UDP Multicast Open.vi"("time-to-live (1)"=u16 5, "multicast addr"=w2, "port"=u16 10000) -> ("error out"=w4:errorcluster, "connection ID"=w5:refnum<k16>)  [unwired: 6 in, 1 out]
  n182 = call-poly <vilib>:"UDP Multicast Open.vi"("time-to-live (1)"=u16 5, "multicast addr"=w30, "port"=u16 10000) -> ("error out"=w32:errorcluster, "connection ID"=w33:refnum<k16>)  [unwired: 6 in, 1 out]
  n183 = String To IP(1:"239.1.4.6" ("name")) -> (0:w44:u32)
  n184 = node-c288() -> (w15:T1)  [unwired: 4 in]
  n185 = String To IP(1:"239.1.4.6" ("name")) -> (0:w1:u32)
  n186 = call-poly <vilib>:"UDP Multicast Open.vi"("time-to-live (1)"=u16 5, "multicast addr"=w44, "port"=u16 10000) -> ("error out"=w46:errorcluster, "connection ID"=w47:refnum<k16>)  [unwired: 6 in, 1 out]
  n187 = node-c288() -> (w43:T1)  [unwired: 4 in]
  n188 = call-poly <vilib>:"UDP Multicast Open.vi"("net address"=w1, "multicast addr"=w1, "port"=u16 10000) -> ("error out"=w59:errorcluster, "connection ID"=w60:refnum<k16>)  [unwired: 6 in, 1 out]
  n189 = String To IP(1:"239.1.4.6" ("name")) -> (0:w16:u32)
  n190 = node-c288() -> (w57:T1)  [unwired: 4 in]
  n191 = call-poly <vilib>:"UDP Multicast Open.vi"("time-to-live (1)"=u16 5, "multicast addr"=w16, "port"=u16 10000) -> ("error out"=w18:errorcluster, "connection ID"=w19:refnum<k16>)  [unwired: 6 in, 1 out]
  n192 = node-c288() -> (w69:T1)  [unwired: 4 in]
  n193 = timed-loop {
    tunnel: w5 -> [w517]
    tunnel: w4 -> [w516]
    timing: w15 -> [_]
    timing-out: [_] -> w14
    shift-right: [w506] -> _
    shift-left: FALSE -> [w509]
    tunnel: [w505] -> w7
    tunnel: [w503] -> w6
    tunnel: [w501] -> _
    tunnel: w2 -> [w500]
    stop <- w502 stop-if-true
    w501 = FALSE
    # "UDP Broadcast loop"
    n194 = node-c288() -> ()  [unwired: 1 in, 1 out]
    n195 = local read "Flight Number 5"() -> (w512:string)
    n196 = feedback-in #1(w512) -> ()
    n197 = feedback #1() -> (w511:string)  [unwired: 1 in]
    n198 = Not Equal?(x=w512, y=w511) -> (x != y?=w510:bool)
    n199 = flat-sequence {
      tunnel: w500 -> [w524]
      tunnel: w516 -> [w525]
      tunnel: w517 -> [w526]
      tunnel: [w526] -> w515
      tunnel: [w525] -> w514
      tunnel: [w524] -> w513
      tunnel: w510 -> [w523]
      tunnel: u16 50001 ("port or service name") -> [w535]
      tunnel: w515 -> [w534]
      tunnel: w514 -> [w533]
      tunnel: w513 -> [w532]
      tunnel: [w531] -> w505
      tunnel: [w530] -> w503
      frame #0 {
        n200 = feedback #2(u32 0) -> (w520:u32)
        n201 = case shown="False" w523 {
          tunnel: w520 -> [w527 _]
          tunnel: [w527 u32 0] -> w519
          frame False {
          }
          frame True {
          }
        }
        "UDP_Pack_num 7" <- w519
        n202 = Increment(x=w519) -> (x+1=w521:u32)
        n203 = feedback-in #2(w521) -> ()
      }
      frame #1 {
        n204 = UDP Write(address=w532, port or service name=w535, connection ID=w534, data in="$CHTSOO01, 77,1449761811,0,0,,0,0,0,174,0,0,0,0.00,23.2,739.6,0,0,0.699,0.716,40.1,1c105014", 8:w533) -> (error out=w530:errorcluster, 3:w531:refnum<k16>)  [unwired: 1 in]
      }
    }
    n205 = Select(t=FALSE, s=w509, f=TRUE) -> (s? t:f=w506:bool)
    "UDP_Out Status 7" <- w506
    n206 = node-c288() -> ()  [unwired: 1 in, 1 out]
    n207 = Unbundle(w503) -> ("status"=w504:bool)  [unwired: 2 out]
    n208 = Compound Arithmetic op=OR(w504, w501) -> (w502:bool)
  }
  n209 = node-c288() -> (w29:T1)  [unwired: 4 in]
  n210 = timed-loop {
    tunnel: w33 -> [w555]
    tunnel: w32 -> [w554]
    timing: w43 -> [_]
    timing-out: [_] -> w42
    shift-right: [w544] -> _
    shift-left: FALSE -> [w547]
    tunnel: [w543] -> w35
    tunnel: [w541] -> w34
    tunnel: [w539] -> _
    tunnel: w30 -> [w538]
    stop <- w540 stop-if-true
    w539 = FALSE
    # "UDP Broadcast loop"
    n211 = node-c288() -> ()  [unwired: 1 in, 1 out]
    n212 = local read "Flight Number 3"() -> (w550:string)
    n213 = feedback-in #3(w550) -> ()
    n214 = feedback #3() -> (w549:string)  [unwired: 1 in]
    n215 = Not Equal?(x=w550, y=w549) -> (x != y?=w548:bool)
    n216 = flat-sequence {
      tunnel: w538 -> [w562]
      tunnel: w554 -> [w563]
      tunnel: w555 -> [w564]
      tunnel: [w564] -> w553
      tunnel: [w563] -> w552
      tunnel: [w562] -> w551
      tunnel: w548 -> [w561]
      tunnel: u16 50001 ("port or service name") -> [w573]
      tunnel: w553 -> [w572]
      tunnel: w552 -> [w571]
      tunnel: w551 -> [w570]
      tunnel: [w569] -> w543
      tunnel: [w568] -> w541
      frame #0 {
        n217 = feedback #4(u32 0) -> (w558:u32)
        n218 = case shown="False" w561 {
          tunnel: w558 -> [w565 _]
          tunnel: [w565 u32 0] -> w557
          frame False {
          }
          frame True {
          }
        }
        "UDP_Pack_num 4" <- w557
        n219 = Increment(x=w557) -> (x+1=w559:u32)
        n220 = feedback-in #4(w559) -> ()
      }
      frame #1 {
        n221 = UDP Write(address=w570, port or service name=w573, connection ID=w572, data in="$TEIOZO01, 77,1449761811,0,0,,0,0,0,174,0,0,0,0.00,23.2,739.6,0,0,0.699,0.716,40.1,1c105014", 8:w571) -> (error out=w568:errorcluster, 3:w569:refnum<k16>)  [unwired: 1 in]
      }
    }
    n222 = Select(t=FALSE, s=w547, f=TRUE) -> (s? t:f=w544:bool)
    "UDP_Out Status 4" <- w544
    n223 = node-c288() -> ()  [unwired: 1 in, 1 out]
    n224 = Unbundle(w541) -> ("status"=w542:bool)  [unwired: 2 out]
    n225 = Compound Arithmetic op=OR(w542, w539) -> (w540:bool)
  }
  n226 = node-c288() -> (w13:T1)  [unwired: 4 in]
  n227 = node-c288() -> (w41:T1)  [unwired: 4 in]
  n228 = timed-loop {
    tunnel: w47 -> [w593]
    tunnel: w46 -> [w592]
    timing: w57 -> [_]
    timing-out: [_] -> w56
    shift-right: [w582] -> _
    shift-left: FALSE -> [w585]
    tunnel: [w581] -> w49
    tunnel: [w579] -> w48
    tunnel: [w577] -> _
    tunnel: w44 -> [w576]
    stop <- w578 stop-if-true
    w577 = FALSE
    # "UDP Broadcast loop"
    n229 = node-c288() -> ()  [unwired: 1 in, 1 out]
    n230 = local read "Flight Number"() -> (w588:string)
    n231 = feedback-in #5(w588) -> ()
    n232 = feedback #5() -> (w587:string)  [unwired: 1 in]
    n233 = Not Equal?(x=w588, y=w587) -> (x != y?=w586:bool)
    n234 = flat-sequence {
      tunnel: w576 -> [w600]
      tunnel: w592 -> [w601]
      tunnel: w593 -> [w602]
      tunnel: [w602] -> w591
      tunnel: [w601] -> w590
      tunnel: [w600] -> w589
      tunnel: w586 -> [w599]
      tunnel: u16 50001 ("port or service name") -> [w611]
      tunnel: w591 -> [w610]
      tunnel: w590 -> [w609]
      tunnel: w589 -> [w608]
      tunnel: [w607] -> w581
      tunnel: [w606] -> w579
      frame #0 {
        n235 = feedback #6(u32 0) -> (w596:u32)
        n236 = case shown="False" w599 {
          tunnel: w596 -> [w603 _]
          tunnel: [w603 u32 0] -> w595
          frame False {
          }
          frame True {
          }
        }
        "UDP_Pack_num 5" <- w595
        n237 = Increment(x=w595) -> (x+1=w597:u32)
        n238 = feedback-in #6(w597) -> ()
      }
      frame #1 {
        n239 = UDP Write(address=w608, port or service name=w611, connection ID=w610, data in="$AL52CO01, 77,1449761811,0,0,,0,0,0,174,0,0,0,0.00,23.2,739.6,0,0,0.699,0.716,40.1,1c105014", 8:w609) -> (error out=w606:errorcluster, 3:w607:refnum<k16>)  [unwired: 1 in]
      }
    }
    n240 = Select(t=FALSE, s=w585, f=TRUE) -> (s? t:f=w582:bool)
    "UDP_Out Status 5" <- w582
    n241 = node-c288() -> ()  [unwired: 1 in, 1 out]
    n242 = Unbundle(w579) -> ("status"=w580:bool)  [unwired: 2 out]
    n243 = Compound Arithmetic op=OR(w580, w577) -> (w578:bool)
  }
  n244 = timed-loop {
    tunnel: w60 -> [w631]
    tunnel: w59 -> [w630]
    timing: w69 -> [_]
    timing-out: [_] -> w68
    shift-right: [w620] -> _
    shift-left: FALSE -> [w623]
    tunnel: [w619] -> w64
    tunnel: [w617] -> w63
    tunnel: [w615] -> _
    tunnel: w1 -> [w614]
    stop <- w616 stop-if-true
    w615 = FALSE
    # "UDP Broadcast loop"
    n245 = node-c288() -> ()  [unwired: 1 in, 1 out]
    n246 = local read "Flight Number"() -> (w626:string)
    n247 = feedback-in #7(w626) -> ()
    n248 = feedback #7() -> (w625:string)  [unwired: 1 in]
    n249 = Not Equal?(x=w626, y=w625) -> (x != y?=w624:bool)
    n250 = flat-sequence {
      tunnel: w614 -> [w638]
      tunnel: w630 -> [w639]
      tunnel: w631 -> [w640]
      tunnel: [w640] -> w629
      tunnel: [w639] -> w628
      tunnel: [w638] -> w627
      tunnel: w624 -> [w637]
      tunnel: u16 50001 ("port or service name") -> [w649]
      tunnel: w629 -> [w648]
      tunnel: w628 -> [w647]
      tunnel: w627 -> [w646]
      tunnel: [w645] -> w619
      tunnel: [w644] -> w617
      frame #0 {
        n251 = feedback #8(u32 0) -> (w634:u32)
        n252 = case shown="False" w637 {
          tunnel: w634 -> [w641 _]
          tunnel: [w641 u32 0] -> w633
          frame False {
          }
          frame True {
          }
        }
        "UDP_Pack_num 3" <- w633
        n253 = Increment(x=w633) -> (x+1=w635:u32)
        n254 = feedback-in #8(w635) -> ()
      }
      frame #1 {
        n255 = UDP Write(address=w646, port or service name=w649, connection ID=w648, data in="$CHFGGA01, 77,1449761811,0,0,,0,0,0,174,0,0,0,0.00,23.2,739.6,0,0,0.699,0.716,40.1,1c105014", 8:w647) -> (error out=w644:errorcluster, 3:w645:refnum<k16>)  [unwired: 1 in]
      }
    }
    n256 = Select(t=FALSE, s=w623, f=TRUE) -> (s? t:f=w620:bool)
    "UDP_Out Status 3" <- w620
    n257 = node-c288() -> ()  [unwired: 1 in, 1 out]
    n258 = Unbundle(w617) -> ("status"=w618:bool)  [unwired: 2 out]
    n259 = Compound Arithmetic op=OR(w618, w615) -> (w616:bool)
  }
  n260 = node-c288() -> (w55:T1)  [unwired: 4 in]
  n261 = node-c288() -> (w62:T1)  [unwired: 4 in]
  n262 = timed-loop {
    tunnel: w19 -> [w669]
    tunnel: w18 -> [w668]
    timing: w29 -> [_]
    timing-out: [_] -> w28
    shift-right: [w658] -> _
    shift-left: FALSE -> [w661]
    tunnel: [w657] -> w21
    tunnel: [w655] -> w20
    tunnel: [w653] -> _
    tunnel: w16 -> [w652]
    stop <- w654 stop-if-true
    w653 = FALSE
    # "UDP Broadcast loop"
    n263 = node-c288() -> ()  [unwired: 1 in, 1 out]
    n264 = local read "Flight Number 4"() -> (w664:string)
    n265 = feedback-in #9(w664) -> ()
    n266 = feedback #9() -> (w663:string)  [unwired: 1 in]
    n267 = Not Equal?(x=w664, y=w663) -> (x != y?=w662:bool)
    n268 = flat-sequence {
      tunnel: w652 -> [w676]
      tunnel: w668 -> [w677]
      tunnel: w669 -> [w678]
      tunnel: [w678] -> w667
      tunnel: [w677] -> w666
      tunnel: [w676] -> w665
      tunnel: w662 -> [w675]
      tunnel: u16 50001 ("port or service name") -> [w687]
      tunnel: w667 -> [w686]
      tunnel: w666 -> [w685]
      tunnel: w665 -> [w684]
      tunnel: [w683] -> w657
      tunnel: [w682] -> w655
      frame #0 {
        n269 = feedback #10(u32 0) -> (w672:u32)
        n270 = case shown="False" w675 {
          tunnel: w672 -> [w679 _]
          tunnel: [w679 u32 0] -> w671
          frame False {
          }
          frame True {
          }
        }
        "UDP_Pack_num 6" <- w671
        n271 = Increment(x=w671) -> (x+1=w673:u32)
        n272 = feedback-in #10(w673) -> ()
      }
      frame #1 {
        n273 = UDP Write(address=w684, port or service name=w687, connection ID=w686, data in="$CABOZO01, 77,1449761811,0,0,,0,0,0,174,0,0,0,0.00,23.2,739.6,0,0,0.699,0.716,40.1,1c105014", 8:w685) -> (error out=w682:errorcluster, 3:w683:refnum<k16>)  [unwired: 1 in]
      }
    }
    n274 = Select(t=FALSE, s=w661, f=TRUE) -> (s? t:f=w658:bool)
    "UDP_Out Status 6" <- w658
    n275 = node-c288() -> ()  [unwired: 1 in, 1 out]
    n276 = Unbundle(w655) -> ("status"=w656:bool)  [unwired: 2 out]
    n277 = Compound Arithmetic op=OR(w656, w653) -> (w654:bool)
  }
  n278 = timed-loop {
    timing: w13 -> [_]
    timing-out: [_] -> w12
    tunnel: w5 -> [w692]
    tunnel: w4 -> [w691]
    stop <- FALSE stop-if-true
    n279 = node-c288() -> ()  [unwired: 1 in, 1 out]
    n280 = UDP Read(connection ID=w692, 8:w691) -> ()  [unwired: 2 in, 5 out]
    n281 = node-c288() -> ()  [unwired: 1 in, 1 out]
  }
  n282 = node-c288() -> (w27:T1)  [unwired: 4 in]
  n283 = timed-loop {
    timing: w41 -> [_]
    timing-out: [_] -> w40
    tunnel: w33 -> [w697]
    tunnel: w32 -> [w696]
    stop <- FALSE stop-if-true
    n284 = node-c288() -> ()  [unwired: 1 in, 1 out]
    n285 = UDP Read(connection ID=w697, 8:w696) -> ()  [unwired: 2 in, 5 out]
    n286 = node-c288() -> ()  [unwired: 1 in, 1 out]
  }
  n287 = timed-loop {
    timing: w55 -> [_]
    timing-out: [_] -> w54
    tunnel: w47 -> [w702]
    tunnel: w46 -> [w701]
    stop <- FALSE stop-if-true
    n288 = node-c288() -> ()  [unwired: 1 in, 1 out]
    n289 = UDP Read(connection ID=w702, 8:w701) -> ()  [unwired: 2 in, 5 out]
    n290 = node-c288() -> ()  [unwired: 1 in, 1 out]
  }
  n291 = timed-loop {
    timing: w62 -> [_]
    timing-out: [_] -> w61
    tunnel: w60 -> [w711]
    tunnel: w59 -> [w710]
    stop <- FALSE stop-if-true
    n292 = node-c288() -> ()  [unwired: 1 in, 1 out]
    n293 = UDP Read(connection ID=w711, 8:w710) -> (data out=→"data out 2":string, error out=→"error out":errorcluster, 4:→"port":u16, 6:→"address":u32)  [unwired: 2 in, 1 out]
    n294 = node-c288() -> ()  [unwired: 1 in, 1 out]
  }
  n295 = timed-loop {
    timing: w27 -> [_]
    timing-out: [_] -> w26
    tunnel: w19 -> [w716]
    tunnel: w18 -> [w715]
    stop <- FALSE stop-if-true
    n296 = node-c288() -> ()  [unwired: 1 in, 1 out]
    n297 = UDP Read(connection ID=w716, 8:w715) -> ()  [unwired: 2 in, 5 out]
    n298 = node-c288() -> ()  [unwired: 1 in, 1 out]
  }
  n299 = node-c288(w12) -> ()  [unwired: 1 out]
  n300 = node-c288(w40) -> ()  [unwired: 1 out]
  n301 = node-c288(w54) -> ()  [unwired: 1 out]
  n302 = node-c288(w61) -> ()  [unwired: 1 out]
  n303 = node-c288(w26) -> ()  [unwired: 1 out]
  n304 = node-c288(w14) -> ()  [unwired: 1 out]
  n305 = node-c288(w42) -> ()  [unwired: 1 out]
  n306 = UDP Close(connection ID=w7, 8:w6) -> (error out=→"UDP_Out_Error Out 7":errorcluster)  [unwired: 1 out]
  n307 = node-c288(w56) -> ()  [unwired: 1 out]
  n308 = UDP Close(connection ID=w35, 8:w34) -> (error out=→"UDP_Out_Error Out 4":errorcluster)  [unwired: 1 out]
  n309 = node-c288(w68) -> ()  [unwired: 1 out]
  n310 = UDP Close(connection ID=w49, 8:w48) -> (error out=→"UDP_Out_Error Out 5":errorcluster)  [unwired: 1 out]
  n311 = UDP Close(connection ID=w64, 8:w63) -> (error out=→"UDP_Out_Error Out 3":errorcluster)  [unwired: 1 out]
  n312 = node-c288(w28) -> ()  [unwired: 1 out]
  n313 = UDP Close(connection ID=w21, 8:w20) -> (error out=→"UDP_Out_Error Out 6":errorcluster)  [unwired: 1 out]
